vi "4Pi Shutter Control.vi"(7 "Calling VI Ref":refnum<vi>) -> ()   [LabVIEW 2016]
uses:
  <vilib>/Utility/miscctls.llb/LVPointTypeDef.ctl
  Hardware Configuration/Hardware Configuration Controls/Device Function.ctl
  Hardware Configuration/Hardware Configuration Controls/Device Type.ctl
  Device Library/Shutters/Shutter Controls/Shutter Actions.ctl
panel:
  in  "Toggle Both":bool
  in  "Quit":bool
  in  "Lower Shutter":bool
  in  "Upper Shutter":bool
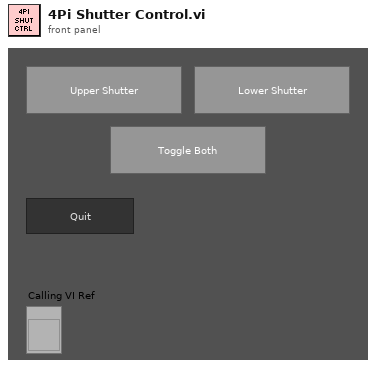
[diagram p1: front panel]
types:
  T1 = enum16{"Always On", "Always Off", "Off While Running"}
  T2 = typedef "LVPointTypeDef.ctl" = cluster{"Horizontal":i16, "Vertical":i16}
  T3 = enum8{"Enabled", "Disabled", "Disabled and Grayed Out"}
  T4 = typedef "Device Function.ctl" = enum16{"Primary", "Secondary", "Overview", "Wide Field Drift Correction", "642 nm Excitation", "560 nm Excitation", "546 nm Excitation", "488 nm Excitation", "405 nm Excitation", "Objective Drift Correction", "Objective XY", "Objective Z", "Sample XY", "Sample Coarse Z", "Sample Z", "4Pi Lower", "4Pi Upper", "Adj Cavity"}
  T5 = typedef "Device Type.ctl" = enum16{"AOTF", "Camera", "Deformable Mirror", "Laser", "Shutter", "Stage"}
  T6 = typedef "Shutter Actions.ctl" = enum16{"Open", "Close", "Toggle", "Status", "Quit"}
  T7 = typedef "LVRectTypeDef.ctl" = cluster{"Left":i16, "Top":i16, "Right":i16, "Bottom":i16}
  T8 = typedef "LVBoundsTypeDef.ctl" = cluster{"Width":u32, "Height":u32}
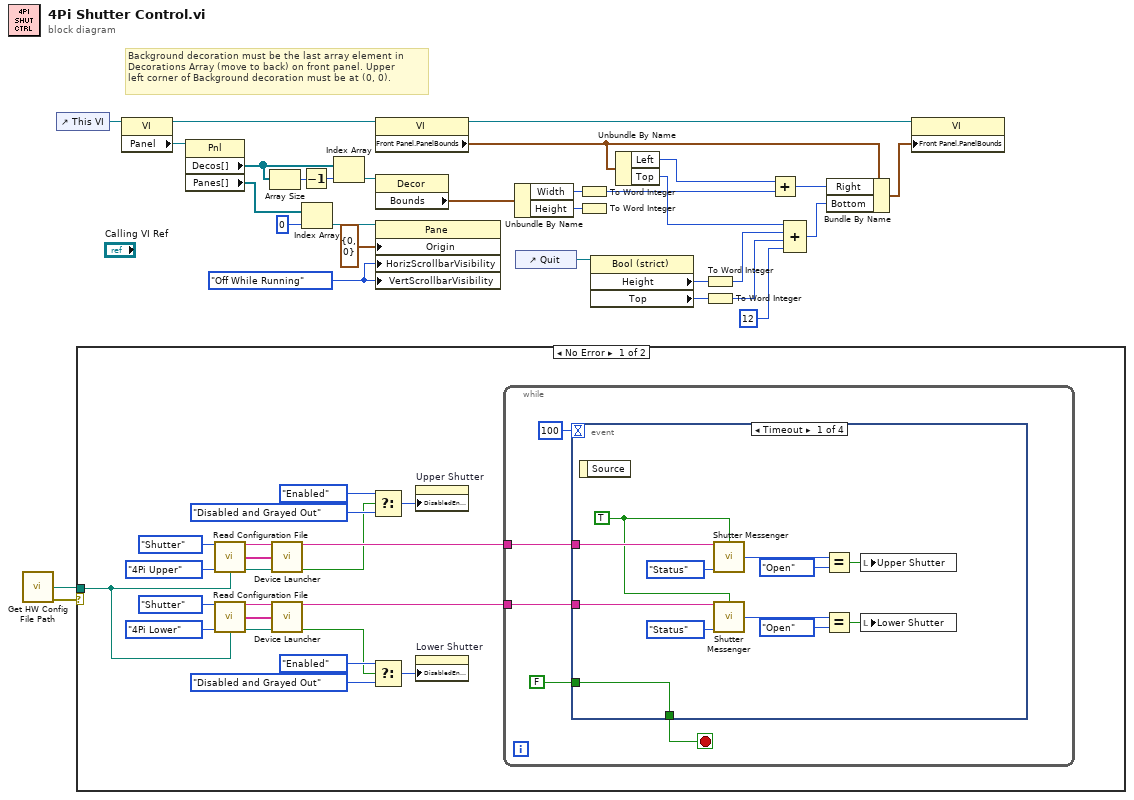
[diagram p0: block diagram]
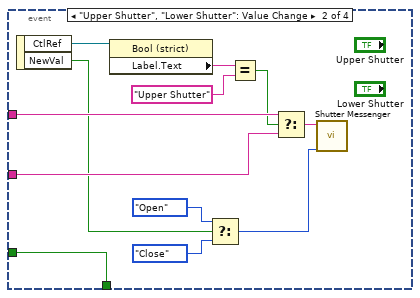
[diagram p2: hidden frame]
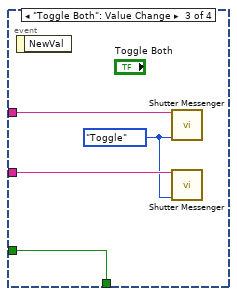
[diagram p3: hidden frame]
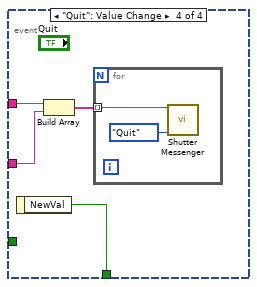
[diagram p4: hidden frame]
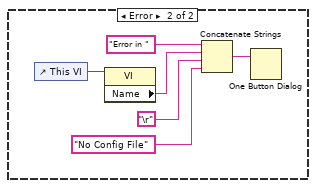
[diagram p5: hidden frame]
diagram:
  w14 = T1."Off While Running" ("Vertical Scrollbar Visibility")
  # "Background decoration must be the last array element in\nDecorations Array (move to back) on front panel. Upper\nleft corner of Background decoration must be at (0, 0)."
  n1 = call "Get HW Config File Path.vi"() -> ("File Path"=w2:path, "Error"=w1:errorcluster)  [unwired: 14 in]
  n2 = control-ref of="This VI"() -> (w7:refnum<vi>)
  n3 = case shown="No Error" w1 {
    tunnel: w2 -> [w34 _]
    frame No Error {
      n4 = call "Read Configuration File.vi"("Device Type"=Device_Type."Shutter", "Device Function"=Device_Function."4Pi Upper", "Config File Path"=w34) -> ("Unique Notifier Name"=w51:string, "Device Ports/IDs/Channels"=w50:string[], "Device Engine Path"=w49:path)  [unwired: 9 in, 1 out]
      n5 = call "Read Configuration File.vi"("Device Type"=Device_Type."Shutter", "Device Function"=Device_Function."4Pi Lower", "Config File Path"=w34) -> ("Unique Notifier Name"=w42:string, "Device Ports/IDs/Channels"=w43:string[], "Device Engine Path"=w44:path)  [unwired: 9 in, 1 out]
      n6 = call "Device Launcher.vi"("Notifier Name"=w51, "Device Ports/IDs/Channels"=w50, "Device Engine Path"=w49) -> ("Notifier Name"=w33:string, "Running?"=w32:bool)  [unwired: 11 in]
      n7 = call "Device Launcher.vi"("Notifier Name"=w42, "Device Ports/IDs/Channels"=w43, "Device Engine Path"=w44) -> ("Notifier Name"=w52:string, "Running?"=w36:bool)  [unwired: 11 in]
      n8 = Select(t=T3."Enabled" ("Disabled"), s=w32, f=T3."Disabled and Grayed Out" ("Disabled")) -> (s? t:f=w39:T3)
      n9 = Select(t=T3."Enabled" ("Disabled"), s=w36, f=T3."Disabled and Grayed Out" ("Disabled")) -> (s? t:f=w35:T3)
      n10 = property on="Upper Shutter" class="Bool (strict)"("DisabledEnum"=w39) -> ()  [unwired: 2 in, 2 out]
      n11 = property on="Lower Shutter" class="Bool (strict)"("DisabledEnum"=w35) -> ()  [unwired: 2 in, 2 out]
      n12 = while {
        tunnel: w33 -> [w56]
        tunnel: w52 -> [w55]
        stop <- w53 stop-if-true
        n13 = event shown="[0] Timeout" {
          selector: _ -> [_ _ _ _]
          dyn-events: _ -> [_ _ _ _]
          timeout: 100 -> [_ _ _ _]
          tunnel: w56 -> [w68 w80 w84 w88]
          tunnel: w55 -> [w67 w79 w83 w87]
          tunnel: FALSE -> [w69 w77 w85 _]
          tunnel: [w69 w77 w85 w89] -> w53
          event Timeout {
            w58 = TRUE ("Quick Status")
            n14 = event-data() -> ()  [unwired: 1 in, 1 out]
            n15 = call "Shutter Messenger.vi"("Notifier Name"=w68, "Quick Status"=w58, "Action"=Shutter_Actions."Status") -> ("Shutter Status"=w64:T6)  [unwired: 11 in, 1 out]
            n16 = call "Shutter Messenger.vi"("Notifier Name"=w67, "Quick Status"=w58, "Action"=Shutter_Actions."Status") -> ("Shutter Status"=w63:T6)  [unwired: 11 in, 1 out]
            n17 = Equal?(x=w64, y=Shutter_Actions."Open") -> (x = y?=w60:bool)
            n18 = Equal?(x=w63, y=Shutter_Actions."Open") -> (x = y?=w59:bool)
            n19 = local write "Upper Shutter"(w60) -> ()
            n20 = local write "Lower Shutter"(w59) -> ()
          }
          event "Upper Shutter", "Lower Shutter": Value Change {
            n21 = event-data() -> ("CtlRef"=w81:refnum<vi>, "NewVal"=w78:bool)  [unwired: 1 in]
            n22 = property class="Bool (strict)"(reference=w81) -> ("Label.Text"=w76:string)  [unwired: 1 in, 2 out]
            n23 = Select(t=Shutter_Actions."Open" ("Action"), s=w78, f=Shutter_Actions."Close" ("Action")) -> (s? t:f=w70:T6)
            n24 = Equal?(x=w76, y="Upper Shutter") -> (x = y?=w74:bool)
            n25 = Select(t=w80, s=w74, f=w79) -> (s? t:f=w73:string)
            n26 = call "Shutter Messenger.vi"("Notifier Name"=w73, "Action"=w70) -> ()  [unwired: 12 in, 2 out]
          }
          event "Toggle Both": Value Change {
            w82 = Shutter_Actions."Toggle" ("Action")
            n27 = event-data() -> ()  [unwired: 1 in, 1 out]
            n28 = call "Shutter Messenger.vi"("Notifier Name"=w84, "Action"=w82) -> ()  [unwired: 12 in, 2 out]
            n29 = call "Shutter Messenger.vi"("Notifier Name"=w83, "Action"=w82) -> ()  [unwired: 12 in, 2 out]
          }
          event "Quit": Value Change {
            n30 = event-data() -> ("NewVal"=w89:bool)  [unwired: 1 in]
            n31 = Build Array(w88, w87) -> (w86:string[])
            n32 = for {
              tunnel: w86 -> [w91] mode=indexing
              n33 = call "Shutter Messenger.vi"("Notifier Name"=w91, "Action"=Shutter_Actions."Quit") -> ()  [unwired: 12 in, 2 out]
            }
          }
        }
      }
    }
    frame Error {
      n34 = control-ref of="This VI"() -> (w97:refnum<vi>)
      n35 = property class="VI"(reference=w97) -> ("Name"=w95:string)  [unwired: 1 in, 2 out]
      n36 = Concatenate Strings("Error in ", w95, "\r", "No Config File") -> (w92:string)
      n37 = One Button Dialog(message=w92) -> ()  [unwired: 1 in, 1 out]
    }
  }
  n38 = property class="VI"(reference=w7) -> (reference out=w15:refnum<vi>, "Panel"=w8:refnum<vi>)  [unwired: 1 in, 1 out]
  n39 = property class="Pnl"(reference=w8) -> ("Decos[]"=w6:refnum<vi>[], "Panes[]"=w11:refnum<vi>[])  [unwired: 1 in, 2 out]
  n40 = Array Size(array=w6) -> (size(s)=w4:i32)
  n41 = Decrement(x=w4) -> (x-1=w5:i32)
  n42 = Index Array(array=w11, index=0) -> (element=w10:refnum<vi>)
  n43 = Index Array(array=w6, index=w5) -> (element=w13:refnum<vi>)
  n44 = property class="VI"(reference=w15) -> (reference out=w17:refnum<vi>, "Front Panel.PanelBounds"=w18:T7)  [unwired: 1 in, 1 out]
  n45 = property class="Decor"(reference=w13) -> ("Bounds"=w16:T8)  [unwired: 1 in, 2 out]
  n46 = property class="Pane"(reference=w10, "Origin"=T2 {"Horizontal"=0, "Vertical"=0}, "HorizScrollbarVisibility"=w14, "VertScrollbarVisibility"=w14) -> ()  [unwired: 1 in, 2 out]
  n47 = Unbundle By Name(w16) -> ("Width"=w21:u32, "Height"=w24:u32)
  n48 = control-ref of="Quit"() -> (w3:refnum<vi>)
  n49 = To Word Integer(number=w21) -> (16bit integer=w23:i16)
  n50 = To Word Integer(number=w24) -> ()  [unwired: 1 out]
  n51 = property class="Bool (strict)"(reference=w3) -> ("Height"=w26:u32, "Top"=w27:i32)  [unwired: 1 in, 2 out]
  n52 = Unbundle By Name(w18) -> ("Left"=w20:i16, "Top"=w31:i16)
  n53 = To Word Integer(number=w26) -> (16bit integer=w29:i16)
  n54 = To Word Integer(number=w27) -> (16bit integer=w30:i16)
  n55 = Add(x=w20, y=w23) -> (x+y=w22:i16)
  n56 = Compound Arithmetic op=ADD(w31, w29, w30, i16 12 ("y")) -> (w25:i16)
  n57 = Bundle By Name(cluster=w18, "Right"=w22, "Bottom"=w25) -> (w19:T7)
  n58 = property class="VI"(reference=w17, "Front Panel.PanelBounds"=w19) -> ()  [unwired: 1 in, 2 out]
